vi "Set Buffer.vi"(6 "Set? [T]":bool=TRUE, 7 "Config in":refnum<class "Carya Config.lvclass">, 8 "error in (no error)":errorcluster, 11 "Carya Config (Buffer) in":refnum<class "CConfig Buffer Type.lvclass">) -> (0 "error out":errorcluster, 2 "Replace?":bool, 3 "Carya Config (Buffer) out":refnum<class "CConfig Buffer Type.lvclass">)   [LabVIEW 2013, in "CConfig Buffer Type.lvclass"]
doc: "Copyright 2018, Carya Automatisering, Wiebe Walstra."
uses:
  CConfig Buffer Type.lvclass
  Carya Config.lvclass
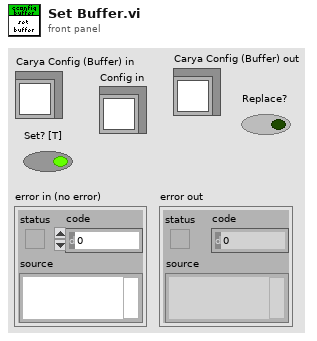
[diagram p1: front panel]
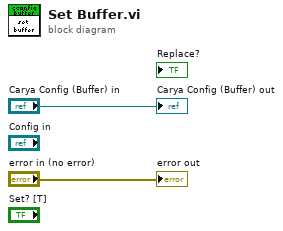
[diagram p0: block diagram]
diagram:
  "error out" <- "error in (no error)"
  "Carya Config (Buffer) out" <- "Carya Config (Buffer) in"
